vi "Interfaz_uart.vi"() -> ()   [LabVIEW 2025]
uses:
  <vilib>/Instr/_visa.llb/VISA Configure Serial Port (Instr).vi
panel:
  in  "Enviar Stats":bool
  in  "Stats":T1={"Engranes"=90.0, "Pulsos"=22, "MAX_RPM"=110}
  in  "Enviar":bool
  in  "Stop Button":bool
  out "Waveform Chart":T2(graph)
  in  "Tab Control":T3(tab)
  out "PWM_num":dbl
  in  "PWM":dbl(slide) scale=0.0..999.0
  in  "Cuad":T4 {"Tiempo en Min" step=10; "Tiempo en Max" step=10}
  in  "Triag":T5
  in  "Diente":T5
  in  "Ramp":T5
  # "ms"
  # "ms"
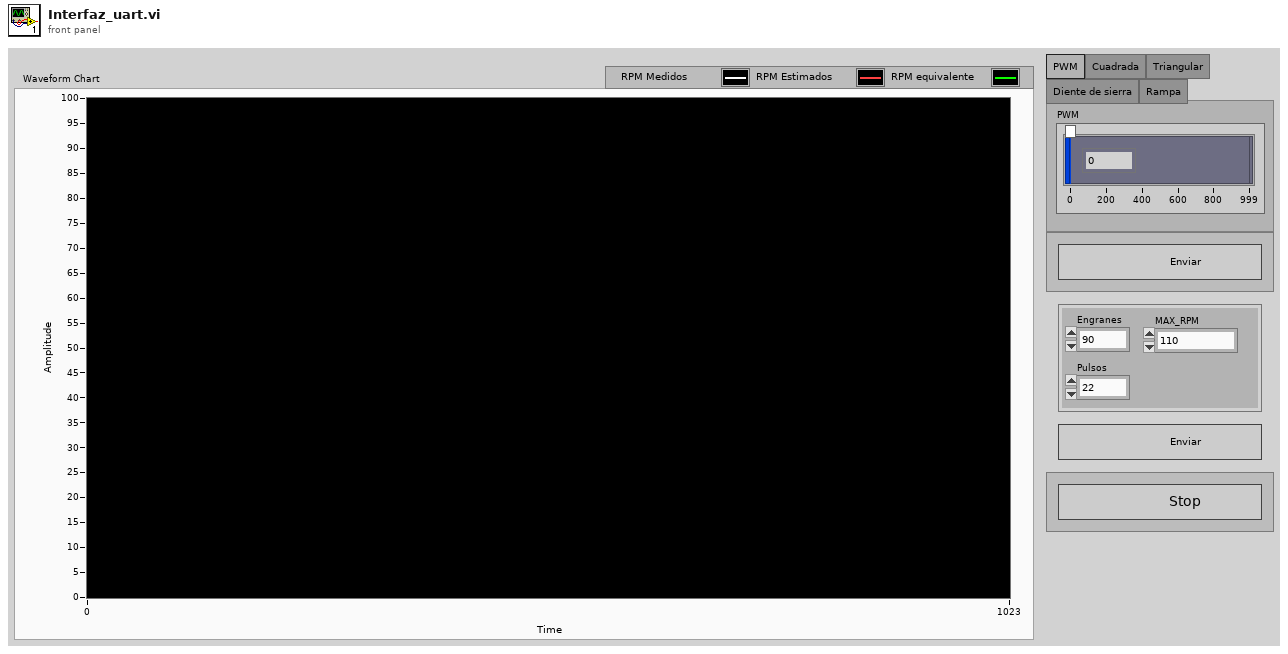
[diagram p1: front panel]
types:
  T1 = cluster{"Engranes":sgl, "Pulsos":u16, "MAX_RPM":u16}
  T2 = cluster{"Número":sgl, "Número":sgl, "Número":sgl}
  T3 = enum32{"PWM", "Cuadrada", "Triangular", "Diente de sierra", "Rampa"}
  T4 = cluster{"Maximo":u16, "Minimo":u16, "Tiempo en Max":u16, "Tiempo en Min":u16}
  T5 = cluster{"Maximo":u16, "Minimo":u16, "Aumento Y":u16, "Aumento X":u16}
  T6 = enum16{"open", "replace", "create", "open or create", "replace or create", "replace or create with confirmation"}
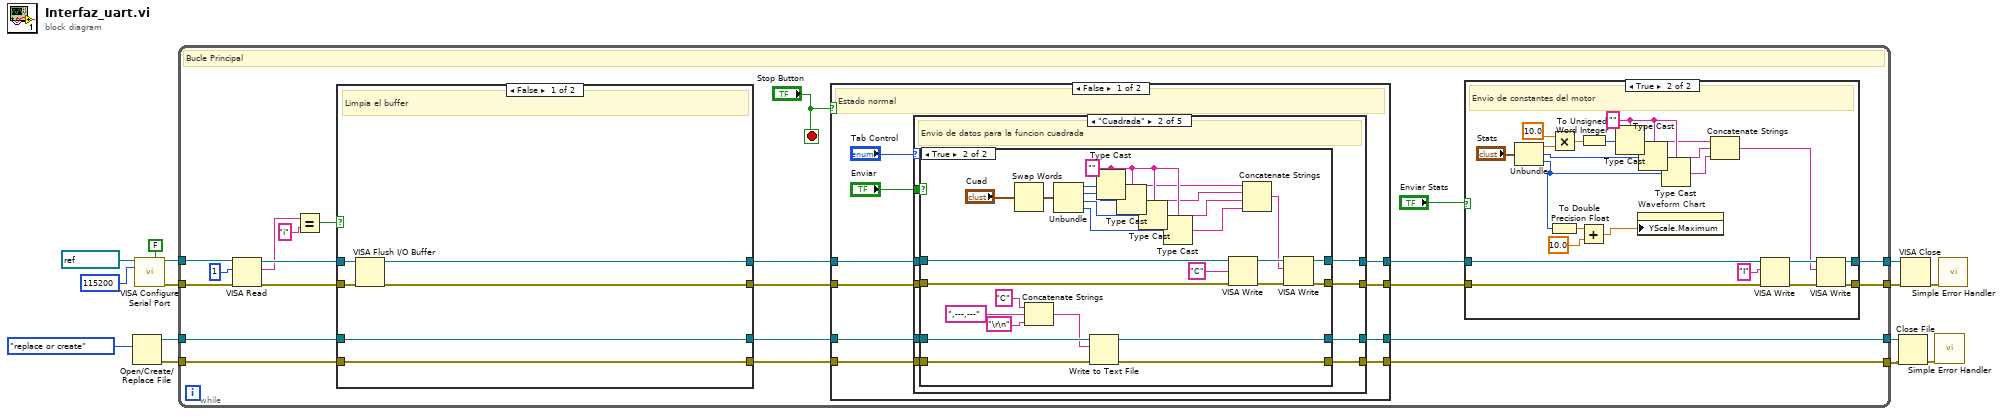
[diagram p0: block diagram]
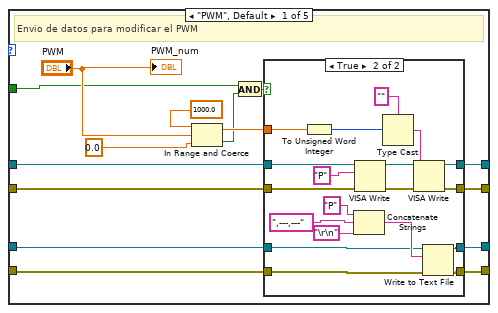
[diagram p3: hidden frame]
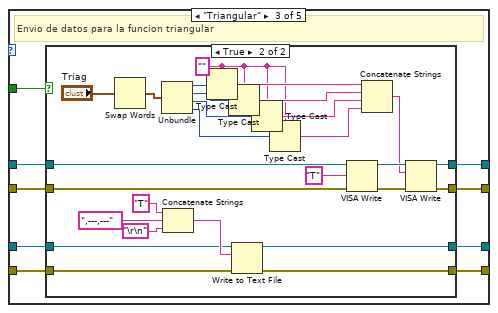
[diagram p6: hidden frame]
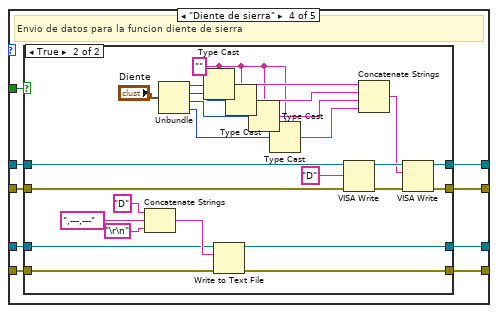
[diagram p8: hidden frame]
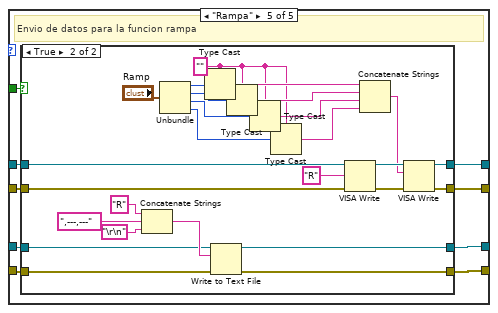
[diagram p10: hidden frame]
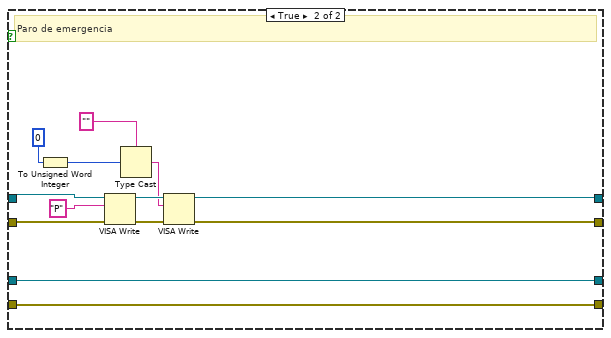
[diagram p12: hidden frame]
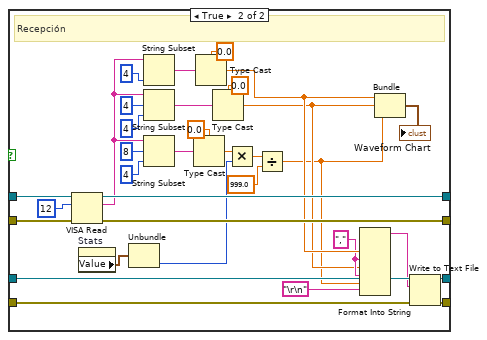
[diagram p13: hidden frame]
diagram:
  n1 = Open/Create/Replace File(operation (0:open)=T6."replace or create") -> (refnum out=w5:refnum<file>, error out=w4:errorcluster)  [unwired: 5 in, 1 out]
  n2 = call-poly "VISA Configure Serial Port"("VISA resource name"=refnum<visa-resource-name> "COM4", "Enable Termination\nChar (T)"=FALSE ("Enable Termination\nChar (T)"), "baud rate (9600)"=u32 115200) -> ("VISA resource name out"=w9:refnum<visa-resource-name>, "error out"=w8:errorcluster)  [unwired: 11 in]
  n3 = while {
    tunnel: w9 -> [w35]
    tunnel: w8 -> [w34]
    tunnel: [w23] -> w14
    tunnel: [w22] -> w13
    tunnel: w5 -> [w20]
    tunnel: w4 -> [w19]
    tunnel: [w16] -> w2
    tunnel: [w15] -> w3
    stop <- "Stop Button" stop-if-true
    # "Bucle Principal"
    n4 = VISA Read(VISA resource name=w35, byte count=u32 1, error in (no error)=w34) -> (VISA resource name out=w33:refnum<visa-resource-name>, read buffer=w31:string, error out=w32:errorcluster)  [unwired: 1 out]
    n5 = Equal?(x=w31, y="i") -> (x = y?=w29:bool)
    n6 = case shown="False" w29 {
      tunnel: [w285 w318] -> w28
      tunnel: [w284 w317] -> w27
      tunnel: w33 -> [w283 w314]
      tunnel: w32 -> [w282 w313]
      tunnel: w20 -> [w281 w299]
      tunnel: w19 -> [w280 w300]
      tunnel: [w281 w298] -> w18
      tunnel: [w280 w297] -> w17
      frame False {
        # "Limpia el buffer"
        n7 = VISA Flush I/O Buffer(VISA resource name=w283, error in (no error)=w282) -> (VISA resource name out=w285:refnum<visa-resource-name>, error out=w284:errorcluster)  [unwired: 1 in]
      }
      frame True {
        w291 = "," ("string")
        # "Recepción"
        n8 = VISA Read(VISA resource name=w314, byte count=u32 12, error in (no error)=w313) -> (VISA resource name out=w318:refnum<visa-resource-name>, read buffer=w306:string, error out=w317:errorcluster)  [unwired: 1 out]
        n9 = property on="Stats" class="Clust (strict)"() -> ("Value"=w287:T1)  [unwired: 2 in, 2 out]
        n10 = Unbundle(w287) -> ("MAX_RPM"=w286:u16)  [unwired: 2 out]
        n11 = String Subset(string=w306, length (rest)=4 ("length (rest)")) -> (substring=w296:string)  [unwired: 1 in]
        n12 = String Subset(string=w306, offset (0)=4, length (rest)=4 ("length (rest)")) -> (substring=w295:string)
        n13 = String Subset(string=w306, offset (0)=8, length (rest)=4 ("length (rest)")) -> (substring=w294:string)
        n14 = Type Cast(type=sgl 0.0 ("Número"), x=w294) -> (*(type *) &x=w304:sgl)
        n15 = Type Cast(type=sgl 0.0 ("Número"), x=w296) -> (*(type *) &x=w292:sgl)
        n16 = Type Cast(type=sgl 0.0 ("Número"), x=w295) -> (*(type *) &x=w290:sgl)
        n17 = Multiply(x=w304, y=w286) -> (x*y=w303:sgl)
        n18 = Divide(x=w303, y=sgl 999.0) -> (x/y=w289:sgl)
        n19 = Format Into String(w292, w291, w290, w291, w289, "\r\n") -> (resulting string=w293:string)  [unwired: 3 in, 1 out]
        n20 = Bundle("Número"=w292, "Número"=w290, w289) -> (→"Waveform Chart":cluster{"Número":sgl, "Número":sgl, sgl})  [unwired: 1 in]
        n21 = Write to Text File(file (use dialog)=w299, text=w293, error in=w300) -> (refnum out=w298:refnum<file>, error out=w297:errorcluster)  [unwired: 1 in, 1 out]
      }
    }
    n22 = case shown="False" "Stop Button" {
      tunnel: w28 -> [w69 w273]
      tunnel: w27 -> [w68 w272]
      tunnel: [w67 w271] -> w25
      tunnel: [w66 w270] -> w24
      tunnel: w18 -> [w64 w268]
      tunnel: w17 -> [w63 w267]
      tunnel: [w62 w268] -> w16
      tunnel: [w61 w267] -> w15
      frame False {
        # "Estado normal"
        n23 = case shown="\"Cuadrada\"" "Tab Control" {
          tunnel: w69 -> [w81 w117 w157 w197 w236]
          tunnel: w68 -> [w80 w116 w156 w196 w235]
          tunnel: [w79 w115 w155 w195 w234] -> w67
          tunnel: [w78 w114 w154 w194 w233] -> w66
          tunnel: "Enviar" -> [w75 w113 w153 w193 w232]
          tunnel: w64 -> [w74 w112 w152 w192 w231]
          tunnel: w63 -> [w73 w111 w151 w191 w230]
          tunnel: [w72 w110 w150 w190 w229] -> w62
          tunnel: [w71 w109 w149 w189 w228] -> w61
          frame "PWM", Default {
            # "Envio de datos para modificar el PWM"
            n24 = In Range and Coerce(upper limit=1000.0, x="PWM", lower limit=0.0) -> (coerced(x)=w85:dbl, In Range?=w84:bool)
            n25 = And(x=w75, y=w84) -> (x .and. y?=w77:bool)
            n26 = case shown="True" w77 {
              tunnel: w81 -> [w89 w108]
              tunnel: w80 -> [w88 w107]
              tunnel: w85 -> [_ w99]
              tunnel: [w89 w103] -> w79
              tunnel: [w88 w102] -> w78
              tunnel: w74 -> [w87 w93]
              tunnel: w73 -> [w86 w92]
              tunnel: [w87 w91] -> w72
              tunnel: [w86 w90] -> w71
              frame False {
              }
              frame True {
                n27 = To Unsigned Word Integer(number=w99) -> (unsigned 16bit integer=w98:u16)
                n28 = Concatenate Strings("P" ("string"), ",---,---" ("text"), "\r\n") -> (w97:string)
                n29 = VISA Write(VISA resource name=w108, write buffer="P", error in (no error)=w107) -> (VISA resource name out=w104:refnum<visa-resource-name>, error out=w105:errorcluster)  [unwired: 1 out]
                n30 = Type Cast(type="", x=w98) -> (*(type *) &x=w101:string)
                n31 = VISA Write(VISA resource name=w104, write buffer=w101, error in (no error)=w105) -> (VISA resource name out=w103:refnum<visa-resource-name>, error out=w102:errorcluster)  [unwired: 1 out]
                n32 = Write to Text File(file (use dialog)=w93, text=w97, error in=w92) -> (refnum out=w91:refnum<file>, error out=w90:errorcluster)  [unwired: 1 in, 1 out]
              }
            }
            "PWM_num" <- "PWM"
          }
          frame "Cuadrada" {
            # "Envio de datos para la funcion cuadrada"
            n33 = case shown="True" w113 {
              tunnel: w117 -> [w121 w148]
              tunnel: w116 -> [w120 w147]
              tunnel: [w121 w144] -> w115
              tunnel: [w120 w143] -> w114
              tunnel: w112 -> [w119 w129]
              tunnel: w111 -> [w118 w128]
              tunnel: [w119 w123] -> w110
              tunnel: [w118 w122] -> w109
              frame False {
              }
              frame True {
                w140 = ""
                n34 = Swap Words(1:"Cuad") -> (0:w130:T4)
                n35 = Concatenate Strings("C" ("string"), ",---,---" ("text"), "\r\n") -> (w124:string)
                n36 = Unbundle(w130) -> ("Maximo"=w142:u16, "Minimo"=w139:u16, "Tiempo en Max"=w138:u16, "Tiempo en Min"=w137:u16)
                n37 = Write to Text File(file (use dialog)=w129, text=w124, error in=w128) -> (refnum out=w123:refnum<file>, error out=w122:errorcluster)  [unwired: 1 in, 1 out]
                n38 = Type Cast(type=w140, x=w142) -> (*(type *) &x=w136:string)
                n39 = Type Cast(type=w140, x=w139) -> (*(type *) &x=w134:string)
                n40 = Type Cast(type=w140, x=w138) -> (*(type *) &x=w133:string)
                n41 = Type Cast(type=w140, x=w137) -> (*(type *) &x=w132:string)
                n42 = VISA Write(VISA resource name=w148, write buffer="C", error in (no error)=w147) -> (VISA resource name out=w145:refnum<visa-resource-name>, error out=w146:errorcluster)  [unwired: 1 out]
                n43 = Concatenate Strings(w136, w134, w133, w132) -> (w135:string)
                n44 = VISA Write(VISA resource name=w145, write buffer=w135, error in (no error)=w146) -> (VISA resource name out=w144:refnum<visa-resource-name>, error out=w143:errorcluster)  [unwired: 1 out]
              }
            }
          }
          frame "Triangular" {
            # "Envio de datos para la funcion triangular"
            n45 = case shown="True" w153 {
              tunnel: w157 -> [w161 w188]
              tunnel: w156 -> [w160 w187]
              tunnel: [w161 w184] -> w155
              tunnel: [w160 w183] -> w154
              tunnel: w152 -> [w159 w165]
              tunnel: w151 -> [w158 w164]
              tunnel: [w159 w163] -> w150
              tunnel: [w158 w162] -> w149
              frame False {
              }
              frame True {
                w171 = ""
                n46 = Swap Words(1:"Triag") -> (0:w173:T5)
                n47 = Unbundle(w173) -> ("Maximo"=w182:u16, "Minimo"=w180:u16, "Aumento Y"=w179:u16, "Aumento X"=w170:u16)
                n48 = Concatenate Strings("T" ("string"), ",---,---" ("text"), "\r\n") -> (w166:string)
                n49 = Type Cast(type=w171, x=w182) -> (*(type *) &x=w178:string)
                n50 = Type Cast(type=w171, x=w180) -> (*(type *) &x=w175:string)
                n51 = Write to Text File(file (use dialog)=w165, text=w166, error in=w164) -> (refnum out=w163:refnum<file>, error out=w162:errorcluster)  [unwired: 1 in, 1 out]
                n52 = Type Cast(type=w171, x=w179) -> (*(type *) &x=w176:string)
                n53 = Type Cast(type=w171, x=w170) -> (*(type *) &x=w172:string)
                n54 = VISA Write(VISA resource name=w188, write buffer="T", error in (no error)=w187) -> (VISA resource name out=w185:refnum<visa-resource-name>, error out=w186:errorcluster)  [unwired: 1 out]
                n55 = Concatenate Strings(w178, w175, w176, w172) -> (w177:string)
                n56 = VISA Write(VISA resource name=w185, write buffer=w177, error in (no error)=w186) -> (VISA resource name out=w184:refnum<visa-resource-name>, error out=w183:errorcluster)  [unwired: 1 out]
              }
            }
          }
          frame "Diente de sierra" {
            # "Envio de datos para la funcion diente de sierra"
            n57 = case shown="True" w193 {
              tunnel: w197 -> [w201 w227]
              tunnel: w196 -> [w200 w226]
              tunnel: [w201 w223] -> w195
              tunnel: [w200 w222] -> w194
              tunnel: w192 -> [w199 w205]
              tunnel: w191 -> [w198 w204]
              tunnel: [w199 w203] -> w190
              tunnel: [w198 w202] -> w189
              frame False {
              }
              frame True {
                w211 = ""
                n58 = Concatenate Strings("D" ("string"), ",---,---" ("text"), "\r\n") -> (w206:string)
                n59 = Unbundle("Diente") -> ("Maximo"=w221:u16, "Minimo"=w219:u16, "Aumento Y"=w218:u16, "Aumento X"=w210:u16)
                n60 = Type Cast(type=w211, x=w221) -> (*(type *) &x=w217:string)
                n61 = Write to Text File(file (use dialog)=w205, text=w206, error in=w204) -> (refnum out=w203:refnum<file>, error out=w202:errorcluster)  [unwired: 1 in, 1 out]
                n62 = Type Cast(type=w211, x=w219) -> (*(type *) &x=w215:string)
                n63 = Type Cast(type=w211, x=w218) -> (*(type *) &x=w214:string)
                n64 = Type Cast(type=w211, x=w210) -> (*(type *) &x=w212:string)
                n65 = VISA Write(VISA resource name=w227, write buffer="D", error in (no error)=w226) -> (VISA resource name out=w224:refnum<visa-resource-name>, error out=w225:errorcluster)  [unwired: 1 out]
                n66 = Concatenate Strings(w217, w215, w214, w212) -> (w216:string)
                n67 = VISA Write(VISA resource name=w224, write buffer=w216, error in (no error)=w225) -> (VISA resource name out=w223:refnum<visa-resource-name>, error out=w222:errorcluster)  [unwired: 1 out]
              }
            }
          }
          frame "Rampa" {
            # "Envio de datos para la funcion rampa"
            n68 = case shown="True" w232 {
              tunnel: w236 -> [w240 w266]
              tunnel: w235 -> [w239 w265]
              tunnel: [w240 w262] -> w234
              tunnel: [w239 w261] -> w233
              tunnel: w231 -> [w238 w244]
              tunnel: w230 -> [w237 w243]
              tunnel: [w238 w242] -> w229
              tunnel: [w237 w241] -> w228
              frame False {
              }
              frame True {
                w249 = ""
                n69 = Concatenate Strings("R" ("string"), ",---,---" ("text"), "\r\n") -> (w245:string)
                n70 = Unbundle("Ramp") -> ("Maximo"=w260:u16, "Minimo"=w258:u16, "Aumento Y"=w257:u16, "Aumento X"=w250:u16)
                n71 = Type Cast(type=w249, x=w260) -> (*(type *) &x=w256:string)
                n72 = Write to Text File(file (use dialog)=w244, text=w245, error in=w243) -> (refnum out=w242:refnum<file>, error out=w241:errorcluster)  [unwired: 1 in, 1 out]
                n73 = Type Cast(type=w249, x=w258) -> (*(type *) &x=w254:string)
                n74 = Type Cast(type=w249, x=w257) -> (*(type *) &x=w253:string)
                n75 = Type Cast(type=w249, x=w250) -> (*(type *) &x=w251:string)
                n76 = VISA Write(VISA resource name=w266, write buffer="R", error in (no error)=w265) -> (VISA resource name out=w263:refnum<visa-resource-name>, error out=w264:errorcluster)  [unwired: 1 out]
                n77 = Concatenate Strings(w256, w254, w253, w251) -> (w255:string)
                n78 = VISA Write(VISA resource name=w263, write buffer=w255, error in (no error)=w264) -> (VISA resource name out=w262:refnum<visa-resource-name>, error out=w261:errorcluster)  [unwired: 1 out]
              }
            }
          }
        }
      }
      frame True {
        # "Paro de emergencia"
        n79 = To Unsigned Word Integer(number=u16 0) -> (unsigned 16bit integer=w276:u16)
        n80 = VISA Write(VISA resource name=w273, write buffer="P", error in (no error)=w272) -> (VISA resource name out=w277:refnum<visa-resource-name>, error out=w278:errorcluster)  [unwired: 1 out]
        n81 = Type Cast(type="", x=w276) -> (*(type *) &x=w275:string)
        n82 = VISA Write(VISA resource name=w277, write buffer=w275, error in (no error)=w278) -> (VISA resource name out=w271:refnum<visa-resource-name>, error out=w270:errorcluster)  [unwired: 1 out]
      }
    }
    n83 = case shown="True" "Enviar Stats" {
      tunnel: w25 -> [w38 w45]
      tunnel: w24 -> [w37 w44]
      tunnel: [w38 w49] -> w23
      tunnel: [w37 w50] -> w22
      frame False {
      }
      frame True {
        w54 = ""
        # "Envio de constantes del motor"
        n84 = Unbundle("Stats") -> ("Engranes"=w59:sgl, "Pulsos"=w55:u16, "MAX_RPM"=w42:u16)
        n85 = Multiply(x=sgl 10.0, y=w59) -> (x*y=w57:sgl)
        n86 = To Double Precision Float(number=w42) -> (double precision float=w41:dbl)
        n87 = To Unsigned Word Integer(number=w57) -> (unsigned 16bit integer=w56:u16)
        n88 = Add(x=w41, y=10.0) -> (x+y=w39:dbl)
        n89 = Type Cast(type=w54, x=w56) -> (*(type *) &x=w53:string)
        n90 = property on="Waveform Chart" class="WFChart (strict)"("YScale.Maximum"=w39) -> ()  [unwired: 2 in, 2 out]
        n91 = Type Cast(type=w54, x=w55) -> (*(type *) &x=w52:string)
        n92 = Type Cast(type=w54, x=w42) -> (*(type *) &x=w51:string)
        n93 = Concatenate Strings(w53, w52, w51) -> (w46:string)
        n94 = VISA Write(VISA resource name=w45, write buffer="I", error in (no error)=w44) -> (VISA resource name out=w48:refnum<visa-resource-name>, error out=w47:errorcluster)  [unwired: 1 out]
        n95 = VISA Write(VISA resource name=w48, write buffer=w46, error in (no error)=w47) -> (VISA resource name out=w49:refnum<visa-resource-name>, error out=w50:errorcluster)  [unwired: 1 out]
      }
    }
  }
  n96 = Close File(refnum=w2, error in=w3) -> (error out=w1:errorcluster)  [unwired: 1 out]
  n97 = VISA Close(VISA resource name=w14, error in (no error)=w13) -> (error out=w7:errorcluster)
  n98 = call <vilib>:"Simple Error Handler.vi"("error in (no error)"=w1) -> ()  [unwired: 4 in, 5 out]
  n99 = call <vilib>:"Simple Error Handler.vi"("error in (no error)"=w7) -> ()  [unwired: 4 in, 5 out]
